vi "Calcular NPS Aplicado.vi"(10 "Rango de MAX de referencia BD":string, 11 "Ponderacion BD":string[](array[string])=["-39.4", "-26.2", "-16.1", "-8.6", "-3.2", "1.2", "1", "-1.1", "-6.6"]) -> (3 "NPS Aplicado":string[](array[string]))   [LabVIEW 2019, in "Prueba33.lvclass"]
uses:
  Prueba33.lvclass
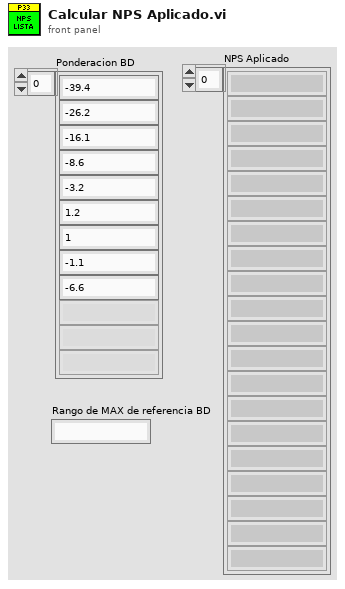
[diagram p1: front panel]
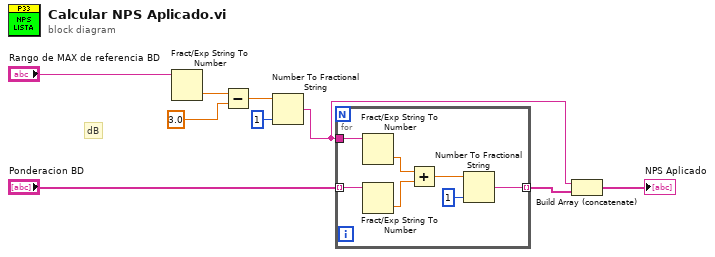
[diagram p0: block diagram]
diagram:
  # "dB"
  n1 = Fract/Exp String To Number(string="Rango de MAX de referencia BD") -> (number=w5:dbl)  [unwired: 3 in, 1 out]
  n2 = Subtract(x=w5, y=3.0) -> (x-y=w3:dbl)
  n3 = Number To Fractional String(number=w3, precision (6)=i16 1) -> (F-format string=w2:string)  [unwired: 2 in]
  n4 = for {
    tunnel: "Ponderacion BD" -> [w15] mode=indexing
    tunnel: w2 -> [w16]
    tunnel: [w10] -> w8 mode=indexing
    n5 = Fract/Exp String To Number(string=w16) -> (number=w14:dbl)  [unwired: 3 in, 1 out]
    n6 = Fract/Exp String To Number(string=w15) -> (number=w13:dbl)  [unwired: 3 in, 1 out]
    n7 = Add(x=w14, y=w13) -> (x+y=w12:dbl)
    n8 = Number To Fractional String(number=w12, precision (6)=i16 1) -> (F-format string=w10:string)  [unwired: 2 in]
  }
  n9 = Build Array (concatenate)(w2, w8) -> (→"NPS Aplicado":string[])
